vi "Get Strain.vi"(6 "Channel":i32, 8 "error in (no error)":errorcluster, 11 "RP100 in":refnum<class "RP100.lvclass">) -> (0 "error out":errorcluster, 2 "Strain (V)":dbl, 3 "RP100 out":refnum<class "RP100.lvclass">)   [LabVIEW 2016, in "RP100.lvclass"]
uses:
  RP100.lvclass
  C:/Program Files (x86)/National Instruments/LabVIEW 2016/user.lib/LevyLab/Levylab Instruments/SMOs/Instrument/Instrument.lvclass
  <userlib>/LevyLab/Levylab Instruments/SMOs/Instrument/Instrument.lvclass/Instrument.ctl
  <userlib>/LevyLab/Levylab Instruments/SMOs/Instrument/Instrument.lvclass
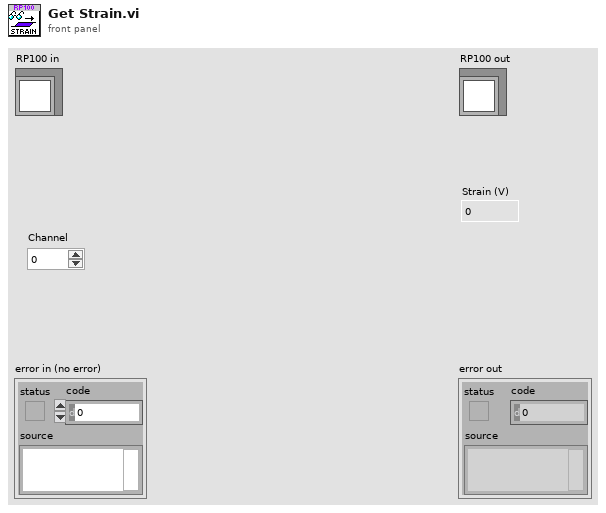
[diagram p1: front panel]
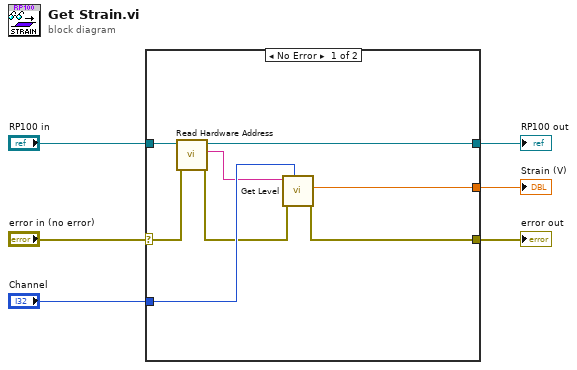
[diagram p0: block diagram]
diagram:
  n1 = case shown="No Error" "error in (no error)" {
    selector: "error in (no error)" -> [w8 w16]
    tunnel: [w10 w16] -> w5
    tunnel: "RP100 in" -> [w14 w15]
    tunnel: [w13 w15] -> w3
    tunnel: "Channel" -> [w12 _]
    tunnel: [w9 _] -> w1
    frame No Error {
      n2 = call <userlib>:"Read Hardware Address.vi"("error in (no error)"=w8, "Instrument in"=w14) -> ("error out"=w7:errorcluster, "Address"=w11:string, "Instrument out"=w13:refnum<class "RP100.lvclass">)  [unwired: 7 in]
      n3 = call "Get Level.vi"("Output Channel"=w12, "error in (no error)"=w7, "VISA resource name"=w11) -> ("error out"=w10:errorcluster, "Level (V"=w9:dbl)  [unwired: 6 in, 1 out]
    }
    frame Error {
    }
  }
  "error out" <- w5
  "RP100 out" <- w3
  "Strain (V)" <- w1
